vi "Write Kasli Alias.vi"(8 "error in (no error)":errorcluster, 10 "Kasli alias":string, 11 "Kasli Wrapper 2.0 in":refnum<class "Kasli Wrapper 2.0.lvclass">) -> (0 "error out":errorcluster, 3 "Kasli Wrapper 2.0 out":refnum<class "Kasli Wrapper 2.0.lvclass">)   [LabVIEW 2020, in "CIRCUS_uServices.lvlib" / "Kasli Wrapper 2.0.lvlib" / "Kasli Wrapper 2.0.lvclass"]
uses:
  Kasli Wrapper 2.0.lvclass
  Kasli Wrapper 2.0.lvclass/Kasli Wrapper 2.0.ctl
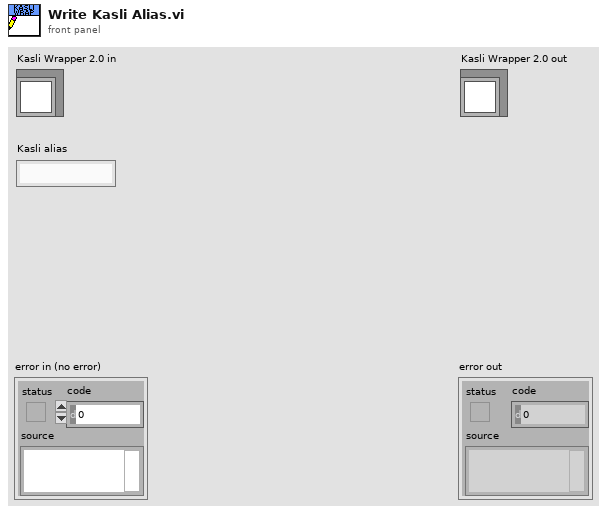
[diagram p1: front panel]
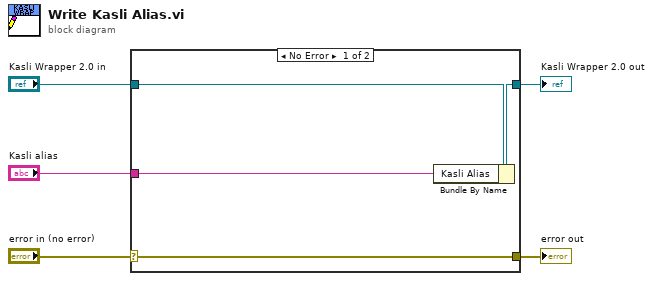
[diagram p0: block diagram]
diagram:
  n1 = case shown="No Error" "error in (no error)" {
    selector: "error in (no error)" -> [w9 w10]
    tunnel: [w9 w10] -> w4
    tunnel: [w7 w11] -> w2
    tunnel: "Kasli Wrapper 2.0 in" -> [w8 w11]
    tunnel: "Kasli alias" -> [w6 _]
    frame No Error {
      n2 = Bundle By Name(cluster=w8, "Kasli Alias"=w6) -> (w7:refnum<class "Kasli Wrapper 2.0.lvclass">)
    }
    frame Error {
    }
  }
  "error out" <- w4
  "Kasli Wrapper 2.0 out" <- w2
